vi "ParseGetFilename.vi"(10 "Length of filemarker":i32, 11 "message in in":string) -> (0 "Filename":string, 3 "data out":string)   [LabVIEW 2023, in "TCP_Server_Connection_Handler.lvlib" / "TCP_Server_Connection_Handler.lvclass"]
uses:
  TCP_Server_Connection_Handler.lvclass
  TCP_Server_Connection_Handler.lvclass/TCP_Server_Connection_Handler.ctl
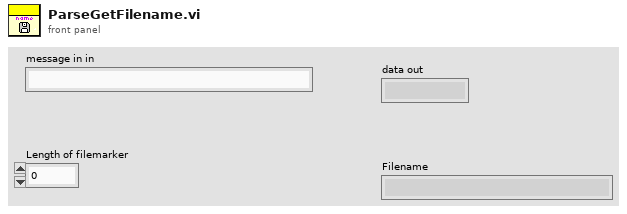
[diagram p1: front panel]
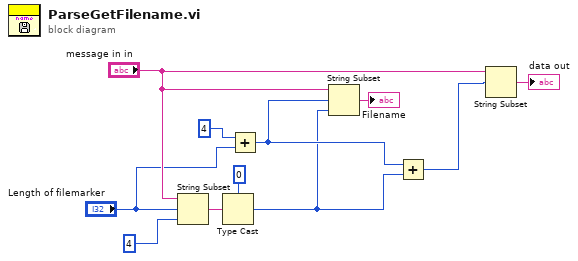
[diagram p0: block diagram]
diagram:
  n1 = String Subset(string="message in in", offset (0)="Length of filemarker", length (rest)=4 ("length (rest)")) -> (substring=w10:string)
  n2 = Type Cast(type=0, x=w10) -> (*(type *) &x=w4:i32)
  n3 = Add(x=4, y="Length of filemarker") -> (x+y=w5:i32)
  n4 = String Subset(string="message in in", offset (0)=w5, length (rest)=w4) -> (substring=→"Filename":string)
  n5 = Add(x=w5, y=w4) -> (x+y=w3:i32)
  n6 = String Subset(string="message in in", offset (0)=w3) -> (substring=→"data out":string)  [unwired: 1 in]
